vi "CMYK to Colour.vi"(0 "Cyan(%)":dbl format="%#_13g", 5 "Magenta(%)":dbl format="%#_13g", 7 "Yellow(%)":dbl format="%#_13g", 9 "Key/Black(%)":dbl format="%#.2g", 11 "error in (no error)":errorcluster) -> (4 "Color":u32(colorbox), 15 "error out":errorcluster)   [LabVIEW 2018, in "Colour Lab.lvlib"]
uses:
  Colour Lab.lvlib
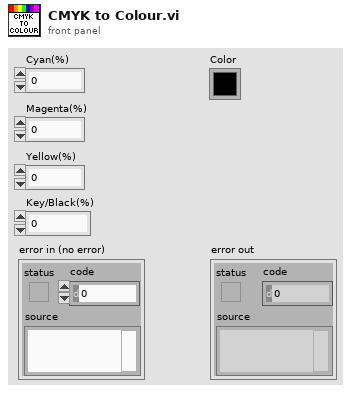
[diagram p1: front panel]
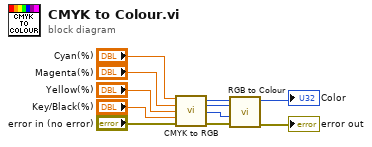
[diagram p0: block diagram]
diagram:
  n1 = call "CMYK to RGB.vi"("Cyan(%)"="Cyan(%)", "Magenta(%)"="Magenta(%)", "Yellow(%)"="Yellow(%)", "Key/Black(%)"="Key/Black(%)", "error in (no error)"="error in (no error)") -> ("Red"=w8:u8, "Green"=w9:u8, "Blue"=w10:u8, "error out"=w11:errorcluster)  [unwired: 7 in]
  n2 = call "RGB to Colour.vi"("error in (no error)"=w11, "Blue"=w10, "Green"=w9, "Red"=w8) -> ("error out"=→"error out":errorcluster, "Color"=→"Color":u32)  [unwired: 6 in]
